vi "PrechargeState.vi"(8 "error in (no error)":errorcluster, 9 "Cluster in":T2, 10 "Enum in":T1, 11 "Actual Start [i]":i64) -> (0 "error out":errorcluster, 2 "Cluster out":T2, 3 "Enum":T1)   [LabVIEW 2018]
uses:
  Type_Def/Type_Def Actuator Controls.ctl
  Type_Def/Type_Def ControlState.ctl
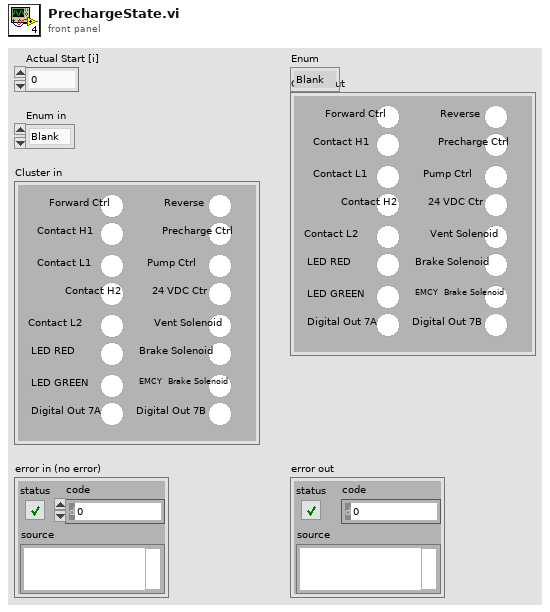
[diagram p1: front panel]
types:
  T1 = typedef "Type_Def ControlState.ctl" = enum16{"Blank", "Systems Check", "Idle", "Ready", "Pushing", "CrawlingPrecharge", "Braking", "Fault", "Boot Up", "Unpowered", "Crawling", "Shutdown", "Service Push", "Service Wait", "Vent", "Precharge"}
  T2 = typedef "Type_Def Actuator Controls.ctl" = cluster{"Reverse ":bool, "Precharge Ctrl":bool, "Pump Ctrl":bool, "24 VDC Ctr":bool, "Vent Solenoid":bool, "Brake Solenoid":bool, "EMCY  Brake Solenoid":bool, "Digital Out 7B ":bool, "Forward Ctrl":bool, "Contact H1":bool, "Contact L1":bool, "Contact H2":bool, "Contact L2 ":bool, "LED RED":bool, "LED GREEN":bool, " Digital Out 7A":bool}
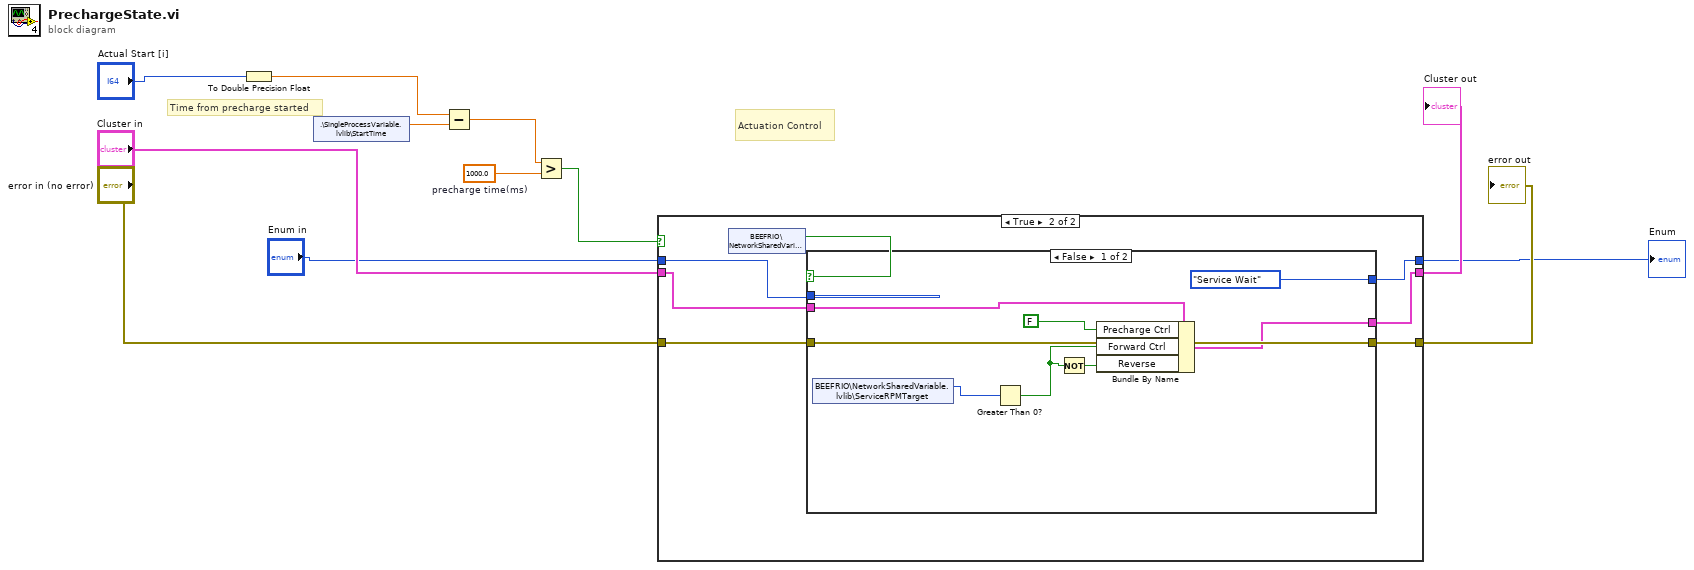
[diagram p0: block diagram]
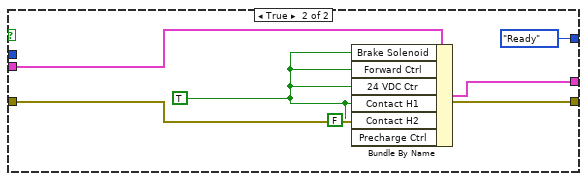
[diagram p3: hidden frame]
diagram:
  w11 = 1000.0  # precharge time(ms)
  # "Time from precharge started"
  # "Actuation Control"
  n1 = To Double Precision Float(number="Actual Start [i]") -> (double precision float=w1:dbl)
  n2 = shared-variable ".\\SingleProcessVariable.lvlib\\StartTime"() -> (w9:dbl)  [unwired: 1 in, 1 out]
  n3 = Subtract(x=w1, y=w9) -> (x-y=w10:dbl)
  n4 = Greater?(x=w10, y=w11) -> (0:w12:bool)
  n5 = case shown="True" w12 {
    tunnel: "Enum in" -> [w15 w22]
    tunnel: [w15 w21] -> w3
    tunnel: "Cluster in" -> [w14 w20]
    tunnel: [w14 w19] -> w5
    tunnel: [w13 w18] -> w6
    tunnel: "error in (no error)" -> [w13 w17]
    frame False {
    }
    frame True {
      n6 = shared-variable "BEEFRIO\\NetworkSharedVariable.lvlib\\Ready"() -> (w16:bool)  [unwired: 1 in, 1 out]
      n7 = case shown="False" w16 {
        tunnel: w22 -> [_ _]
        tunnel: [Type_Def_ControlState."Service Wait" Type_Def_ControlState."Ready"] -> w21
        tunnel: w20 -> [w28 w35]
        tunnel: [w27 w34] -> w19
        tunnel: [w30 w33] -> w18
        tunnel: w17 -> [w30 w33]
        frame False {
          n8 = shared-variable "BEEFRIO\\NetworkSharedVariable.lvlib\\ServiceRPMTarget"() -> (w25:i16)  [unwired: 1 in, 1 out]
          n9 = Greater Than 0?(x=w25) -> (x > 0?=w24:bool)
          n10 = Not(x=w24) -> (.not. x?=w23:bool)
          n11 = Bundle By Name(cluster=w28, "Precharge Ctrl"=FALSE, "Forward Ctrl"=w24, "Reverse"=w23) -> (w27:T2)
        }
        frame True {
          w31 = TRUE
          n12 = Bundle By Name(cluster=w35, "Brake Solenoid"=w31, "Forward Ctrl"=w31, "24 VDC Ctr"=w31, "Contact H1"=w31, "Contact H2"=w31, "Precharge Ctrl"=FALSE) -> (w34:T2)
        }
      }
    }
  }
  "error out" <- w6
  "Cluster out" <- w5
  "Enum" <- w3
